vi "Send 1 Scan.vi"(0 "Connection ID in":refnum<k5>, 5 "Port":T2, 11 "error in (no error)":errorcluster) -> (3 "Out of Range":bool, 4 "Connection ID out":refnum<k5>, 6 "voltage data":sgl format="%.5f", 8 "Scaled data":sgl format="%.2f", 10 "Output Cluster":T1 {"scaled" format="%.2f"; "voltage" format="%.2f"}, 12 "units":string, 14 "Time":dbl format="%.2f", 15 "error out":errorcluster)   [LabVIEW 2012]
uses:
  DataServer/command cluster.ctl
  DataServer/command.ctl
  DataServer/data send.ctl
  DAQ configuration/channel identifier.ctl
  DAQ configuration/sensor cluster.ctl
  calibration/global scale array.vi
panel:
  in  "data":T3 {"seconds since 1904" format="%.2f"; "voltage data" format="%.4f"}
  out "data out":T4 {"arbitrary time (s)" format="%.2f"; "voltage data" format="%.5f"}
  in  "command interface":T5={"command"=enum."Idle", "start time (ms)"=0, "Channel Indices"=[], "Scans per Sample"=1} {"Scans per Sample" min=1}
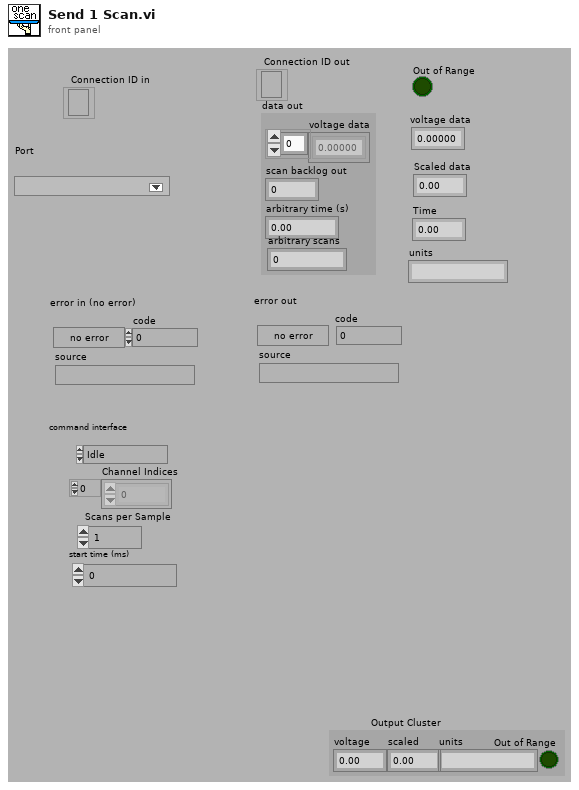
[diagram p1: front panel]
types:
  T1 = typedef "sensor cluster.ctl" = cluster{"voltage":sgl, "scaled":sgl, "units":string, "Out of Range":bool}
  T2 = typedef "channel identifier.ctl" = u16
  T3 = typedef "data send.ctl" = cluster{"voltage data":sgl[], "scan backlog":u32, "seconds since 1904":dbl, "arbitrary scans":i32}
  T4 = cluster{"voltage data":sgl[], "scan backlog out":u32, "arbitrary time (s)":dbl, "arbitrary scans":i32}
  T5 = typedef "command cluster.ctl" = cluster{"command":T6, "start time (ms)":u32, "Channel Indices":i32[], "Scans per Sample":i32}
  T6 = typedef "command.ctl" = enum16{"Idle", "Send Data", "Send 1 Scan", "Logoff"}
  T7 = enum16{"Standard", "Buffered", "CRLF", "Immediate"}
  T8 = enum16{"Idle", "Send Data", "Send 1 Scan", "Logoff"}
  T9 = typedef "calib array.ctl" = T10[]
  T10 = typedef "conversion.ctl" = cluster{"conversion matrix":sgl[][], "units":string, "name":string, "scale type":T11, "offset (volts)":dbl, "second channel":i8, "correspondence table":T12, "offset (physical units)":dbl, "pH scale":T13, "D.O.":T14}
  T11 = typedef "scale type.ctl" = enum16{"Volts", "Polynomial", "Correspondence Table", "pH", "Dissolved Oxygen", "Quadratic"}
  T12 = typedef "correspondence table.ctl" = cluster{"physical units":dbl, "volts":dbl}[]
  T13 = typedef "pH scale.ctl" = cluster{"Buffers":cluster{"Buffer":dbl, "Calibrated":bool, "V/T":dbl}[], "Temperature":dbl}
  T14 = typedef "DO scale.ctl" = cluster{"Temperature":dbl, "K":dbl, "barometric pressure":dbl}
  T15 = cluster{"voltage":sgl, sgl, "units":string, "Out of Range":bool}
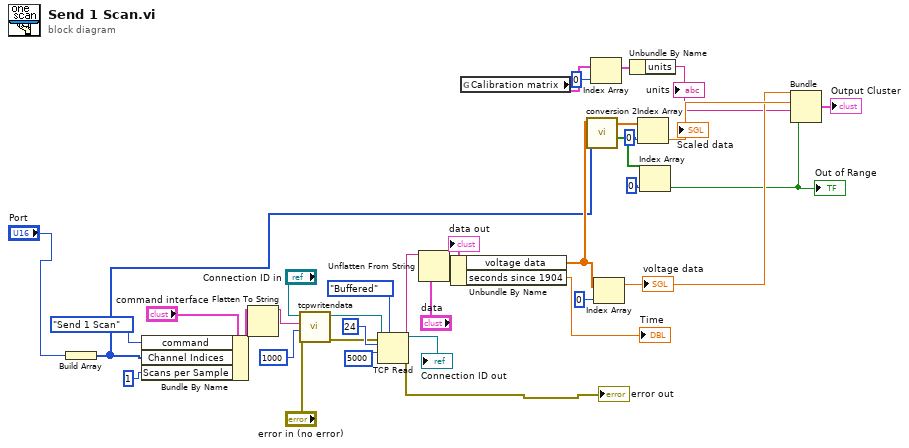
[diagram p0: block diagram]
diagram:
  n1 = Build Array("Port") -> (w10:T2[])
  n2 = Bundle By Name(cluster="command interface", "command"=T8."Send 1 Scan", "Channel Indices"=w10, "Scans per Sample"=1) -> (w32:T5)
  n3 = Flatten To String(anything=w32) -> (data string=w34:string)  [unwired: 3 in, 2 out]
  n4 = call "tcpwritendata.vi"("error in (no error)"="error in (no error)", "timeout ms (25000)"=1000, "data in"=w34, "refnum in"="Connection ID in") -> ("error out"=w15:errorcluster, "refnum out"=w16:refnum<k5>)  [unwired: 5 in, 1 out]
  n5 = TCP Read(connection ID=w16, bytes to read=24 ("y"), error in (no error)=w15, 7:T7."Buffered" ("mode (standard)"), 9:5000 ("timeout ms (25000)")) -> (connection ID out=→"Connection ID out":refnum<k5>, data out=w25:string, error out=→"error out":errorcluster)
  n6 = Unflatten From String(type="data", binary string=w25) -> (value=w19:T3)  [unwired: 3 in, 2 out]
  "data out" <- w19
  n7 = Unbundle By Name(w19) -> ("voltage data"=w22:sgl[], "seconds since 1904"=→"Time":dbl)
  n8 = global read "global scale array.vi" "Calibration matrix"() -> (w8:T9)
  n9 = call "conversion 2.vi"("Channel Indices"=w10, "voltage data"=w22) -> ("Out of Range"=w3:bool[], "calibrated data"=w17:sgl[])  [unwired: 8 in]
  n10 = Index Array(array=w8, index=0 ("Index")) -> (element=w6:T10)
  n11 = Index Array(array=w22, index=0 ("Index")) -> (element=w12:sgl)
  "voltage data" <- w12
  n12 = Unbundle By Name(w6) -> ("units"=w5:string)
  "units" <- w5
  n13 = Index Array(array=w17, index=0 ("Index")) -> (element=w18:sgl)
  "Scaled data" <- w18
  n14 = Index Array(array=w3, index=0 ("Index")) -> (element=w2:bool)
  "Out of Range" <- w2
  n15 = Bundle("voltage"=w12, w18, "units"=w5, "Out of Range"=w2) -> (→"Output Cluster":T15)  [unwired: 1 in]
